vi "Switch Configuration - Topology Event.vi"(8 "error in (no error)":errorcluster, 10 "Topology":string, 11 "Switch Config UI Data in":T1 {"Switch Config Page Item Ref" format="%.0x"}) -> (0 "error out":errorcluster, 3 "Switch Config UI Data Out":T1 {"Switch Config Page Item Ref" format="%.0x"})   [LabVIEW 2015, in "DMM-SWITCH-ScanList System Explorer.lvlib"]
uses:
  DMM-SWITCH-ScanList System Explorer.lvlib
  Configuration Controls/Switch Config VI UI Data.ctl
  Configuration Controls/Switch Config VI UI Ctrl Values.ctl
  Configuration Controls/Switch Config VI UI Ctrl References.ctl
  <instrlib>/niSwitch/niSwitch.LLB/niSwitch Topologies.ctl
  <vilib>/NI Veristand/Custom Device API/Custom Device Item Ref.ctl
  <vilib>/NI Veristand/Custom Device API/Custom Device API.lvlib
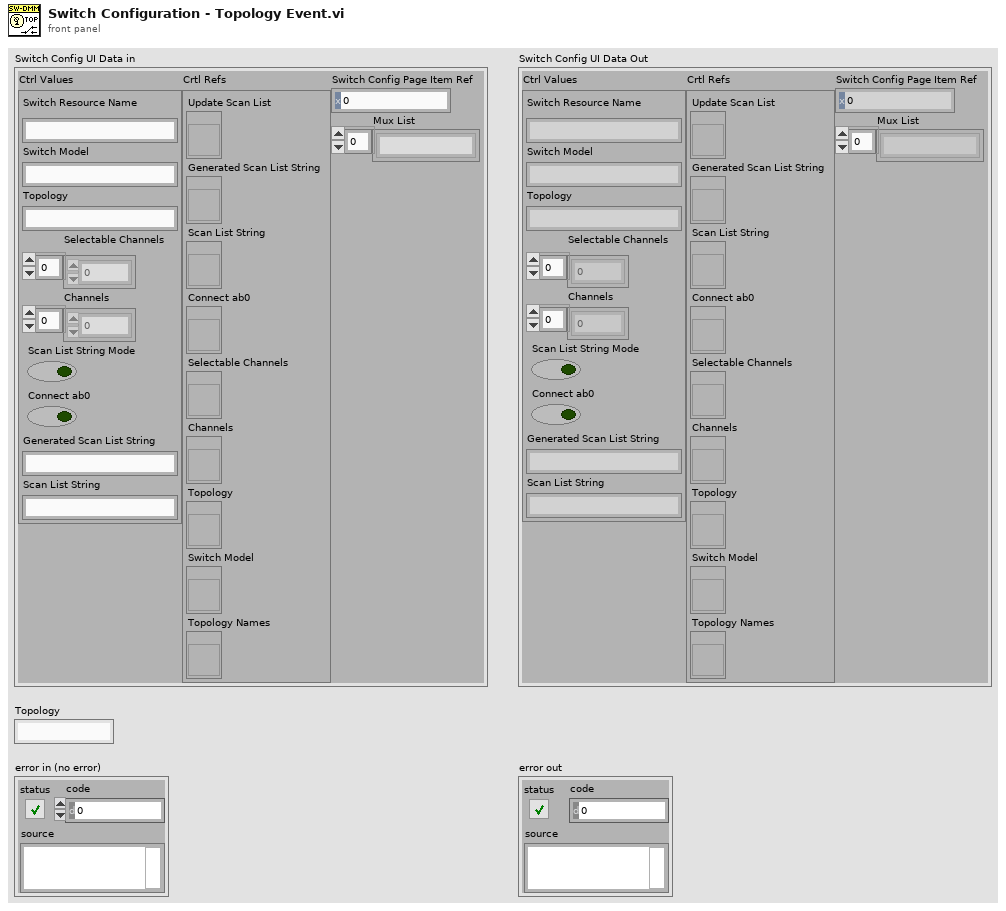
[diagram p1: front panel]
types:
  T1 = typedef "DMM-SWITCH-ScanList System Explorer.lvlib/Switch Config VI UI Data.ctl" = cluster{"Ctrl Values":T2, "Crtl Refs":T3, "Switch Config Page Item Ref":T4, "Mux List":string[]}
  T2 = typedef "DMM-SWITCH-ScanList System Explorer.lvlib/Switch Config VI UI Ctrl Values.ctl" = cluster{"Switch Resource Name":string, "Switch Model":string, "Topology":string, "Selectable Channels":i32[], "Channels":i32[], "Scan List String Mode":bool, "Connect ab0":bool, "Generated Scan List String":string, "Scan List String":string}
  T3 = typedef "DMM-SWITCH-ScanList System Explorer.lvlib/Switch Config VI UI Ctrl References.ctl" = cluster{"Update Scan List":refnum<vi>, "Generated Scan List String":refnum<vi>, "Scan List String":refnum<vi>, "Connect ab0":refnum<vi>, "Selectable Channels":refnum<vi>, "Channels":refnum<vi>, "Topology":refnum<vi>, "Switch Model":refnum<vi>, "Topology Names":refnum<vi>}
  T4 = typedef "Custom Device API.lvlib/Custom Device Item Ref.ctl" = u64
  T5 = enum8{"Enabled", "Disabled", "Disabled and Grayed Out"}
  T6 = typedef "DMM-SWITCH-ScanList System Explorer.lvlib/Topology Data.ctl" = cluster{"Switch Model":string, "Wire Configuration":enum16{"1-Wire", "2-Wire", "4-Wire"}, "Banks Configuration":enum16{"Single", "Dual", "Quad", "Octal", "Sixteen"}, "# of Channels":u32, "Terminated?":bool}
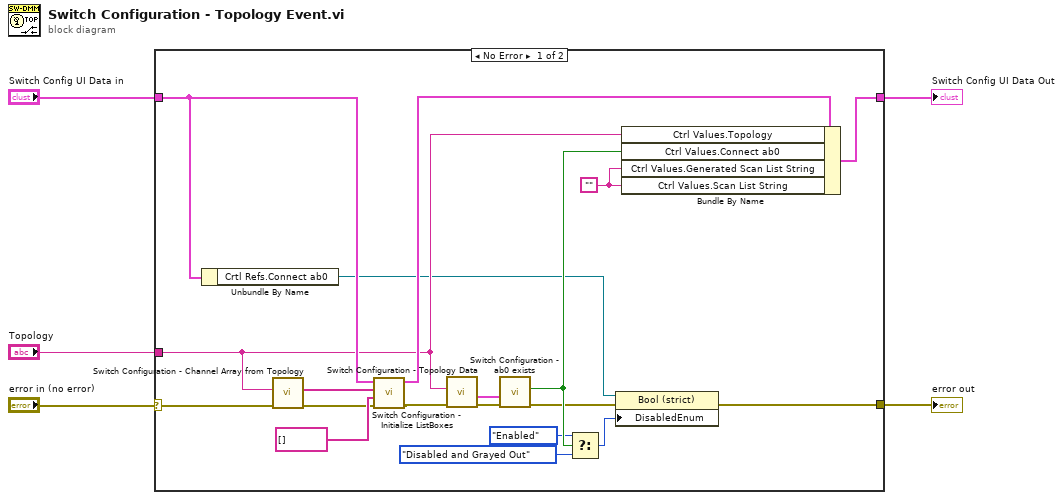
[diagram p0: block diagram]
diagram:
  n1 = case shown="No Error" "error in (no error)" {
    selector: "error in (no error)" -> [w6 w26]
    tunnel: "Switch Config UI Data in" -> [w22 w25]
    tunnel: [w19 w25] -> w4
    tunnel: "Topology" -> [w17 _]
    tunnel: [w15 w26] -> w2
    frame No Error {
      w24 = ""
      n2 = Unbundle By Name(w22) -> ("Crtl Refs.Connect ab0"=w16:refnum<vi>)
      n3 = call "Switch Configuration - Channel Array from Topology.vi"("error in (no error)"=w6, "Selected Mux Topology"=w17) -> ("error out"=w7:errorcluster, "Channel Array Out"=w20:string[])  [unwired: 8 in]
      n4 = call "Switch Configuration - Initialize ListBoxes.vi"("error in (no error)"=w7, "Channels ListBox Items"=string[] [], "Selectable Channels ListBox Items"=w20, "Switch Config UI Data In"=w22) -> ("error out"=w14:errorcluster, "Switch Config UI Data Out"=w23:T1)  [unwired: 6 in]
      n5 = call "Switch Configuration - Topology Data.vi"("error in (no error)"=w14, "Mux Topology"=w17) -> ("error out"=w8:errorcluster, "Topology Data"=w9:T6)  [unwired: 8 in]
      n6 = call "Switch Configuration - ab0 exists.vi"("error in (no error)"=w8, "Topology Data"=w9) -> ("error out"=w10:errorcluster, "ab0 Exists?"=w18:bool)  [unwired: 8 in]
      n7 = Select(t=T5."Enabled" ("Disabled"), s=w18, f=T5."Disabled and Grayed Out" ("Disabled")) -> (s? t:f=w13:T5)
      n8 = property class="Bool (strict)"(reference=w16, error in=w10, "DisabledEnum"=w13) -> (error out=w15:errorcluster)  [unwired: 1 out]
      n9 = Bundle By Name(cluster=w23, "Ctrl Values.Topology"=w17, "Ctrl Values.Connect ab0"=w18, "Ctrl Values.Generated Scan List String"=w24, "Ctrl Values.Scan List String"=w24) -> (w19:T1)
    }
    frame Error {
    }
  }
  "Switch Config UI Data Out" <- w4
  "error out" <- w2
